vi "Operation Selection.VI"(1 "selector":string) -> (0 "result":bool)   [LabVIEW 2017, in "NI_Gmath.lvlib"]
uses:
  <vilib>/gmath/NI_Gmath.lvlib
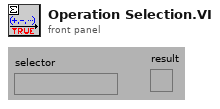
[diagram p1: front panel]
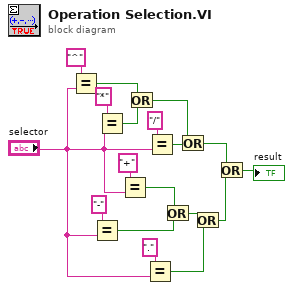
[diagram p0: block diagram]
diagram:
  n1 = Equal?(x="^", y="selector") -> (x = y?=w7:bool)
  n2 = Equal?(x="-", y="selector") -> (x = y?=w10:bool)
  n3 = Equal?(x="*", y="selector") -> (x = y?=w13:bool)
  n4 = Equal?(x="+", y="selector") -> (x = y?=w6:bool)
  n5 = Or(x=w7, y=w13) -> (x .or. y?=w11:bool)
  n6 = Equal?(x=".", y="selector") -> (x = y?=w3:bool)
  n7 = Equal?(x="/", y="selector") -> (x = y?=w12:bool)
  n8 = Or(x=w6, y=w10) -> (x .or. y?=w2:bool)
  n9 = Or(x=w11, y=w12) -> (x .or. y?=w9:bool)
  n10 = Or(x=w2, y=w3) -> (x .or. y?=w1:bool)
  n11 = Or(x=w9, y=w1) -> (x .or. y?=→"result":bool)
